vi "Blur.vi"(0 "image in":refnum<class "MSC Image.lvclass">, 1 "BlurX":i32=3, 2 "BlurY":i32=3, 5 "error in (no error)":errorcluster) -> (14 "image out":refnum<class "MSC Image.lvclass">, 19 "error out":errorcluster)   [LabVIEW 2016, in "MSC Image.lvclass"]
doc: "Blurs the image."
uses:
  MSC Image.lvclass
  Dependencies/x86/MSC I Process32.dll
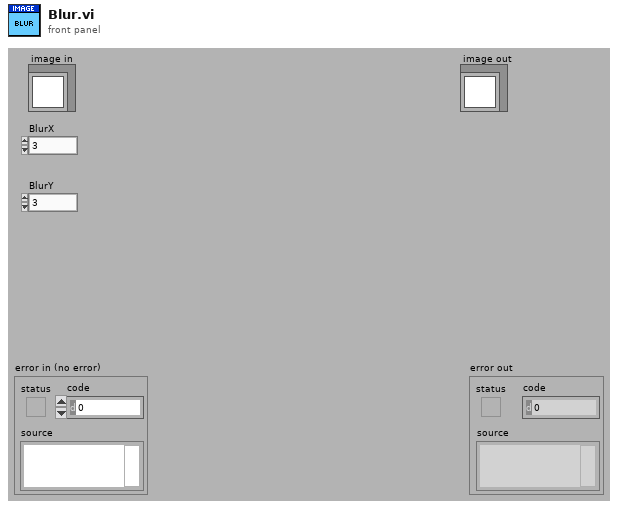
[diagram p1: front panel]
types:
  T1 = typedef "Image.ctl" = cluster{"Pointer":u64, "Size":T2, "Image Type":T3, "Time Stamp":timestamp, "Variant":variant}
  T2 = typedef "Size.ctl" = cluster{"Cols":i32, "Rows":i32}
  T3 = typedef "Image Type.ctl" = i32
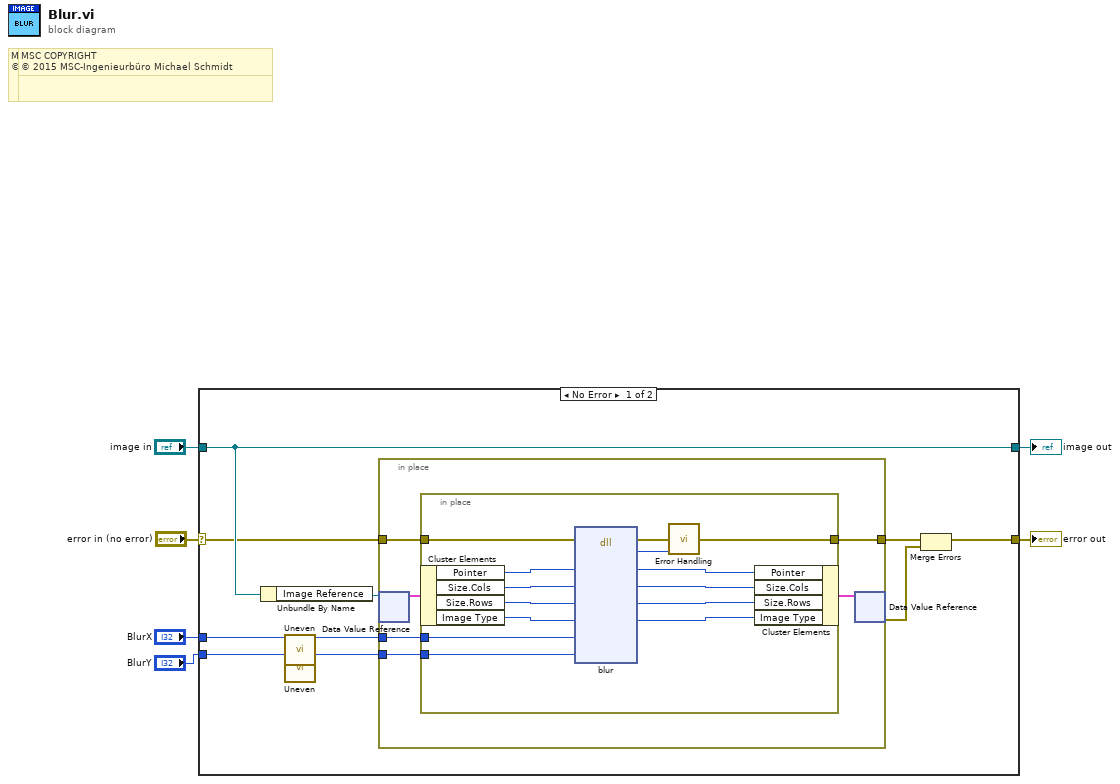
[diagram p0: block diagram]
diagram:
  # "MSC COPYRIGHT\n© 2016 MSC-Ingenieurbüro Michael Schmidt"
  # "MSC COPYRIGHT\n© 2016 MSC-Ingenieurbüro Michael Schmidt"
  # "MSC COPYRIGHT\n© 2015 MSC-Ingenieurbüro Michael Schmidt"
  # "MSC COPYRIGHT\n© 2015 MSC-Ingenieurbüro Michael Schmidt"
  n1 = case shown="No Error" "error in (no error)" {
    selector: "error in (no error)" -> [w12 w38]
    tunnel: [w11 w38] -> w5
    tunnel: [w16 w37] -> w3
    tunnel: "image in" -> [w16 w37]
    tunnel: "BlurX" -> [w10 _]
    tunnel: "BlurY" -> [w8 _]
    frame No Error {
      n2 = Unbundle By Name(w16) -> ("Image Reference"=w15:refnum<data-value>)
      n3 = call "Uneven.vi"("number in"=w10) -> ("uneven number out"=w9:i32)  [unwired: 14 in]
      n4 = call "Uneven.vi"("number in"=w8) -> ("uneven number out"=w7:i32)  [unwired: 14 in]
      n5 = in-place {
        in-place-border: w12 -> [w20]
        in-place-border: [w19] -> w14
        in-place-border: w9 -> [w18]
        in-place-border: w7 -> [w17]
        n6 = in-place-dvr #1(w15) -> (w21:T1)  [unwired: 1 out]
        n7 = in-place {
          in-place-border: w20 -> [w35]
          in-place-border: [w36] -> w19
          in-place-border: w18 -> [w24]
          in-place-border: w17 -> [w23]
          n8 = in-place-cluster #2(w21) -> ("Pointer"=w32:u64, "Size.Cols"=w31:i32, "Size.Rows"=w30:i32, "Image Type"=w29:T3)
          n9 = dll-call lib="C:/Users/MSC/LabVIEW Projekte/LV 2014/MSC I-Process/user.lib/MSC-I Process/Dependencies/x86/MSC I Process*.dll" fn="blur"(error in=w35, "pointer"=w32, "cols"=w31, "rows"=w30, "type"=w29, "blurCols"=w24, "blurRows"=w23) -> (error out=w34:errorcluster, "error"=w33:i32, "pointer"=w25:u64, "cols"=w26:i32, "rows"=w27:i32, "type"=w28:i32)  [unwired: 4 in, 1 out]
          n10 = call "Error Handling.vi"("error in (no error)"=w34, "return type"=w33) -> ("error out"=w36:errorcluster)  [unwired: 12 in, 1 out]
          n11 = in-place-cluster #2("Pointer"=w25, "Size.Cols"=w26, "Size.Rows"=w27, "Image Type"=w28) -> (w22:T1)
        }
        n12 = in-place-dvr #1(w22) -> (w13:errorcluster)  [unwired: 1 out]
      }
      n13 = Merge Errors(w14, w13) -> (w11:errorcluster)
    }
    frame Error {
    }
  }
  "error out" <- w5
  "image out" <- w3
